vi "Date Time Str Converter BAP3B.vi"() -> (2 "String Output":string)   [LabVIEW 2014]
doc: "Date Time Str Converter BAP3B\n\nConverts date and time into a string that can be a file path.\n\nBeverly Abadines\nPHY 350\nBAP3P"
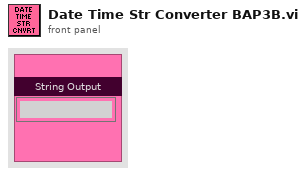
[diagram p1: front panel]
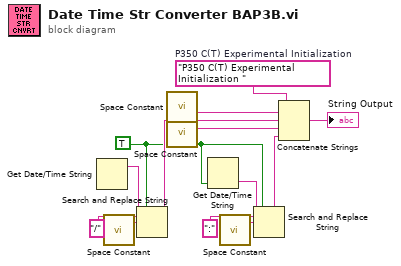
[diagram p0: block diagram]
diagram:
  w2 = TRUE ("want seconds? (F)")
  w4 = "P350 C(T) Experimental Initialization "  # P350 C(T) Experimental Initialization
  n1 = Get Date/Time String() -> (date string=w9:string)  [unwired: 1 in, 3 out]
  n2 = call <vilib>:"Space Constant.vi"() -> ("String"=w7:string)
  n3 = Search and Replace String(replace all?=w2, input string=w9, search string="/", replace string=w7) -> (result string=w10:string)  [unwired: 4 in, 3 out]
  n4 = call <vilib>:"Space Constant.vi"() -> ("String"=w11:string)
  n5 = call <vilib>:"Space Constant.vi"() -> ("String"=w13:string)
  n6 = Get Date/Time String(want seconds? (F)=w2) -> (time string=w3:string)  [unwired: 3 out]
  n7 = call <vilib>:"Space Constant.vi"() -> ("String"=w6:string)
  n8 = Search and Replace String(replace all?=w2, input string=w3, search string=":", replace string=w6) -> (result string=w12:string)  [unwired: 4 in, 3 out]
  n9 = Concatenate Strings(w4, w11, w10, w13, w12) -> (→"String Output":string)
